vi "Engaging.vi"(6 "PID Cluster":T2={"L1 to L4 PID Cluster"={"L1 PID Gains"={"Kp"=0.005, "Kd"=0.5, "Ki"=0.0005}, "L2 PID Gains"={"Kp"=0.01, "Kd"=1.0, "Ki"=0.005}, "L3 PID Gains"={"Kp"=0.05, "Kd"=1.0, "Ki"=0.0005}, "L4 PID Gains"={"Kp"=0.1, "Kd"=0.1, "Ki"=0.0005}}, "Stage PID Cluster"={"Stage Z PID"={"Kp"=0.0005, "Kd"=0.001, "Ki"=0.0}, "Stage Y PID"={"Kp"=0.0003, "Kd"=0.01, "Ki"=0.0}, "Stage X PID"={"Kp"=0.0003, "Kd"=0.01, "Ki"=0.0}}, "OCT Z PID Gains"={"Kp"=0.0003, "Kd"=0.0001, "Ki"=0.01}}, 7 "Offset Home 2 RCM":dbl[](array[numeric])=[0.0, 0.0, 0.0, 0.0], 8 "error in":errorcluster, 9 "Engage Pt":dbl[](array[numeric])=[0.0, 0.0, 0.0, 0.0], 10 "Prev Posit Cluster":T3={"Prev L1 to L4 Posit"=[0.0, 0.0, 0.0, 0.0], "Prev Stage Posit"=[6.0, 6.0, 6.0], "Prev OCT Z Posit"=0.0}, 11 "FPGA VI Reference In":refnum<k20>) -> (0 "error out":errorcluster, 2 "Last Posit Cluster":T1={"Last L1 to L4 Posit"=[0.0, 0.0, 0.0, 0.0], "Last Stage Posit"=[6.0, 6.0, 6.0], "Last OCT Z Posit"=0.0}, 3 "FPGA VI Reference Out":refnum<k20>)   [LabVIEW 2016]
uses:
  <vilib>/Platform/TimedLoop/XDataNode/timing_clust.ctl
  <vilib>/Platform/TimedLoop/XDataNode/nitl_modes.ctl
  <vilib>/Platform/TimedLoop/XDataNode/wakeup.ctl
  Global Variables.vi
  <vilib>/platform/TimedLoop/XDataNode/XDataNode.xnode
  <vilib>/Platform/TimedLoop/XDataNode/XDNodeRunTimeDep.lvlib
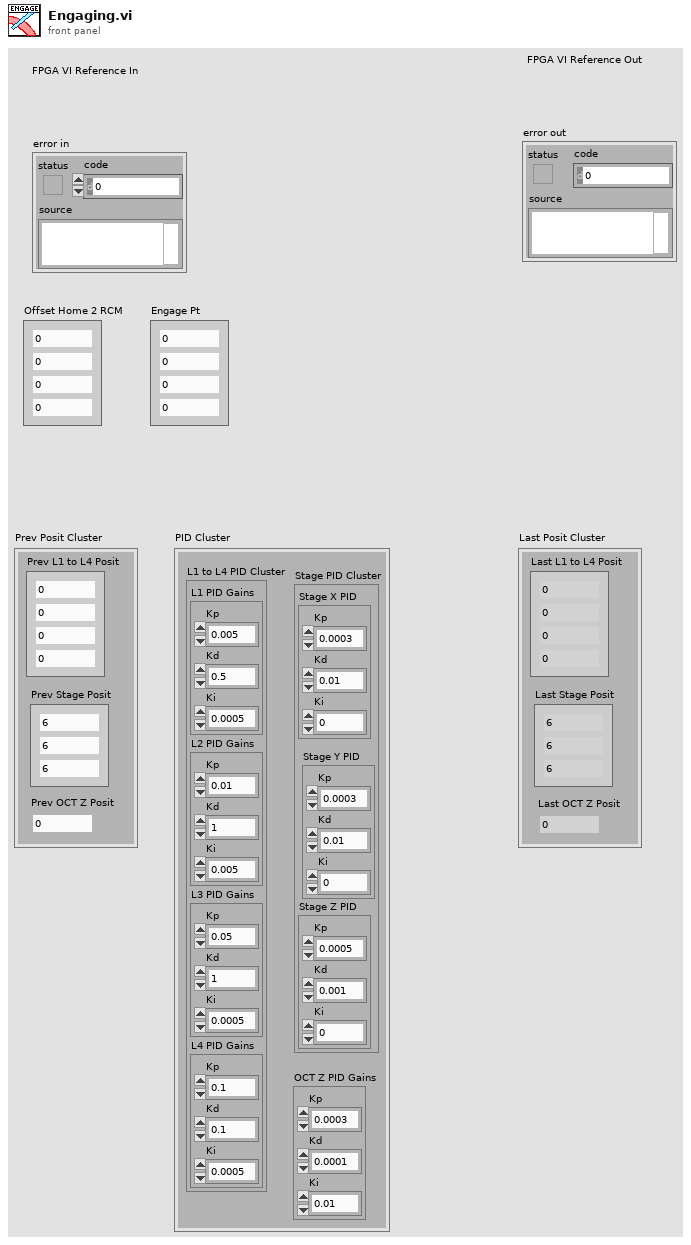
[diagram p1: front panel]
types:
  T1 = cluster{"Last L1 to L4 Posit":dbl[], "Last Stage Posit":dbl[], "Last OCT Z Posit":dbl}
  T2 = cluster{"L1 to L4 PID Cluster":cluster{"L1 PID Gains":cluster{"Kp":dbl, "Kd":dbl, "Ki":dbl}, "L2 PID Gains":cluster{"Kp":dbl, "Kd":dbl, "Ki":dbl}, "L3 PID Gains":cluster{"Kp":dbl, "Kd":dbl, "Ki":dbl}, "L4 PID Gains":cluster{"Kp":dbl, "Kd":dbl, "Ki":dbl}}, "Stage PID Cluster":cluster{"Stage Z PID":cluster{"Kp":dbl, "Kd":dbl, "Ki":dbl}, "Stage Y PID":cluster{"Kp":dbl, "Kd":dbl, "Ki":dbl}, "Stage X PID":cluster{"Kp":dbl, "Kd":dbl, "Ki":dbl}}, "OCT Z PID Gains":cluster{"Kp":dbl, "Kd":dbl, "Ki":dbl}}
  T3 = cluster{"Prev L1 to L4 Posit":dbl[], "Prev Stage Posit":dbl[], "Prev OCT Z Posit":dbl}
  T4 = cluster{"Stop Vacuum":bool, "Vacuum Force":i8, "Max Limit [mmHg]":dbl, "Slide in":i8, "Irrigation?":bool}
  T5 = typedef "XDNodeRunTimeDep.lvlib/timing_clust.ctl" = cluster{"Expected End [f-1]":u64, "Actual End [f-1]":u64, "Finished Late? [f-1]":bool, "Expected End [i-1]":u64, "Actual End [i-1]":u64, "Finished Late? [i-1]":bool, "Expected Start [i]":u64, "Actual Start [i]":u64, "Expected Start [f]":u64, "Actual Start [f]":u64, "Source Name":string, "Structure Name":string, "Period":i64, "Deadline":i64, "Offset":i64, "Start":i64, "Priority":i32, "Timeout":i32, "Mode":T6, "Wakeup Reason":T7, "Error":errorcluster, "Source Type":string, "Secondary Source Type":string, "Global End Time":u64, "Global Start Time":u64, "Frame Duration":u64, "Iteration Duration":u64, "Assigned CPU":i32, "I/O Scan Engine Mode":u32}
  T6 = typedef "XDNodeRunTimeDep.lvlib/nitl_modes.ctl" = enum32{"No Change", "Process missed periods, maintain original phase", "Discard missed periods, maintain original phase", "Process missed periods, ignore original phase", "Discard missed periods, ignore original phase"}
  T7 = typedef "XDNodeRunTimeDep.lvlib/wakeup.ctl" = enum32{"Normal", "Aborted", "Asynchronous wakeup", "Timing source error", "Timed loop error", "Timeout"}
  T8 = cluster{"Stage Z PID":cluster{"Kp":dbl, "Kd":dbl, "Ki":dbl}, "Stage Y PID":cluster{"Kp":dbl, "Kd":dbl, "Ki":dbl}, "Stage X PID":cluster{"Kp":dbl, "Kd":dbl, "Ki":dbl}}
  T9 = cluster{"L1 PID Gains":cluster{"Kp":dbl, "Kd":dbl, "Ki":dbl}, "L2 PID Gains":cluster{"Kp":dbl, "Kd":dbl, "Ki":dbl}, "L3 PID Gains":cluster{"Kp":dbl, "Kd":dbl, "Ki":dbl}, "L4 PID Gains":cluster{"Kp":dbl, "Kd":dbl, "Ki":dbl}}
  T10 = cluster{"Accurus button":bool[], "Accurus engaged?":bool, "Vacuum Force":i32, "Accurus Ch. A Vout":dbl, "Accurus Ch. B Vout":dbl, "Irrigation engaged?":bool}
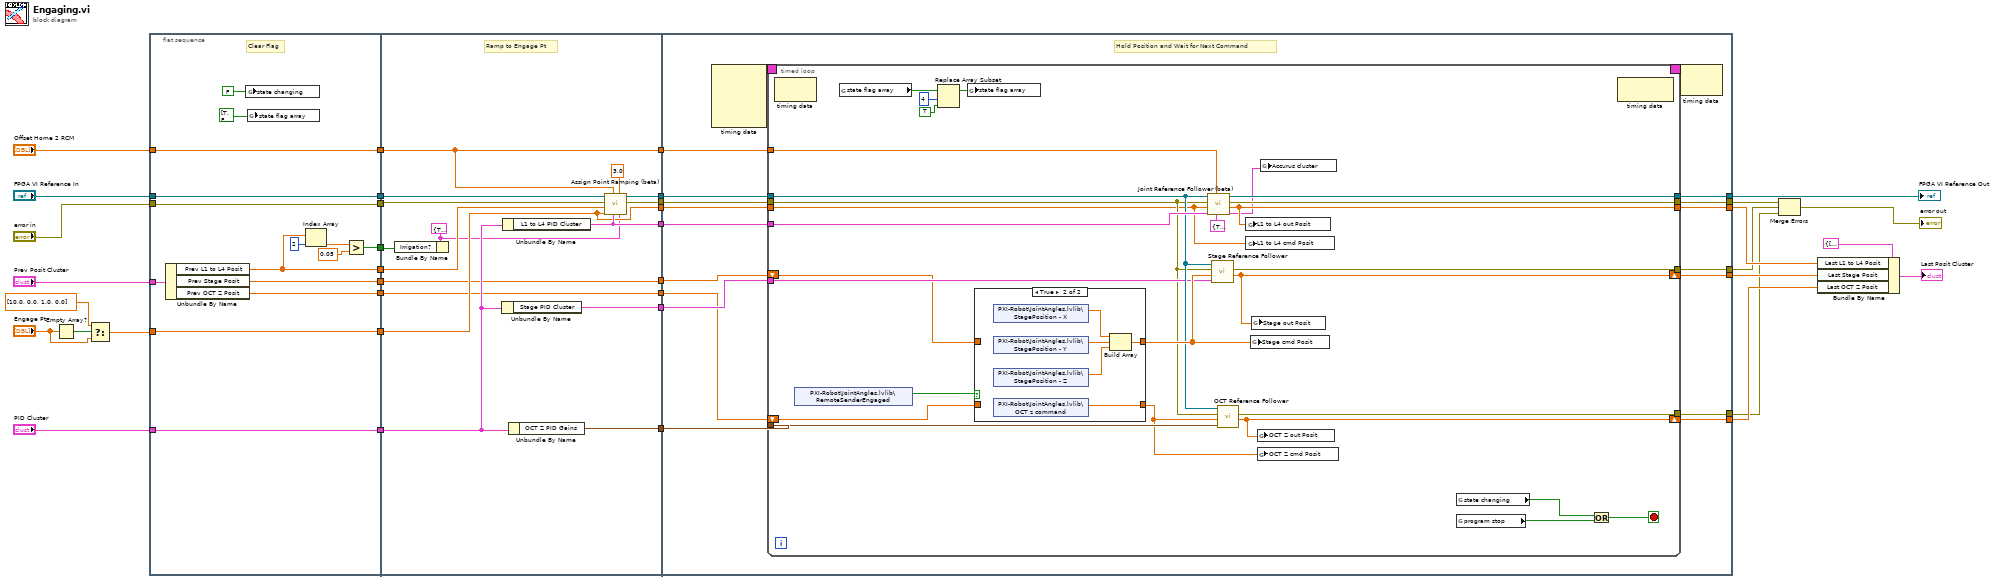
[diagram p0: block diagram]
diagram:
  n1 = Empty Array?(array="Engage Pt") -> (empty?=w29:bool)
  n2 = Select(t=dbl[] [10.0, 0.0, 1.0, 0.0] ("First Trk Pt 2"), s=w29, f="Engage Pt") -> (s? t:f=w26:dbl[])
  n3 = flat-sequence {
    tunnel: [w50] -> w37
    tunnel: "FPGA VI Reference In" -> [w50]
    tunnel: "error in" -> [w49]
    tunnel: [w49] -> w36
    tunnel: [w39] -> w35
    tunnel: "PID Cluster" -> [w47]
    tunnel: "Offset Home 2 RCM" -> [w48]
    tunnel: [w48] -> w33
    tunnel: [w43] -> w31
    tunnel: w26 -> [w43]
    tunnel: [w47] -> w19
    tunnel: "Prev Posit Cluster" -> [w46]
    tunnel: [w45] -> w5
    tunnel: [w44] -> w2
    tunnel: [w38] -> w1
    tunnel: w37 -> [w68]
    tunnel: w36 -> [w67]
    tunnel: w35 -> [w65]
    tunnel: w33 -> [w62]
    tunnel: w31 -> [w57]
    tunnel: [w64] -> w30
    tunnel: [w57] -> w25
    tunnel: [w63] -> w24
    tunnel: [w62] -> w23
    tunnel: [w61] -> w22
    tunnel: w19 -> [w59]
    tunnel: [w60] -> w18
    tunnel: [w58] -> w17
    tunnel: w5 -> [w56]
    tunnel: [w56] -> w4
    tunnel: [w55] -> w3
    tunnel: w2 -> [w55]
    tunnel: w1 -> [w54]
    tunnel: [w80] -> w13
    tunnel: [w79] -> w8
    tunnel: w30 -> [w83]
    tunnel: w25 -> [w82]
    tunnel: w24 -> [w84]
    tunnel: w23 -> [w71]
    tunnel: w22 -> [w81]
    tunnel: [w78] -> w20
    tunnel: [w77] -> w21
    tunnel: w18 -> [w76]
    tunnel: w17 -> [w75]
    tunnel: [w74] -> w14
    tunnel: [w73] -> w7
    tunnel: [w72] -> w6
    tunnel: w4 -> [w70]
    tunnel: w3 -> [w69]
    frame #0 {
      # "Clear Flag"
      n4 = Unbundle By Name(w46) -> ("Prev L1 to L4 Posit"=w39:dbl[], "Prev Stage Posit"=w45:dbl[], "Prev OCT Z Posit"=w44:dbl)
      n5 = global write "Global Variables.vi" "state changing"(FALSE ("state changing")) -> ()
      n6 = global write "Global Variables.vi" "state flag array"(bool[] [TRUE, FALSE, FALSE, FALSE, FALSE, FALSE, FALSE, FALSE, FALSE] ("state flag array")) -> ()
      n7 = Index Array(array=w39, index=2) -> (element=w41:dbl)
      n8 = Greater?(x=w41, y=0.05) -> (0:w38:bool)
    }
    frame #1 {
      w53 = T4 {"Stop Vacuum"=TRUE, "Vacuum Force"=0, "Max Limit [mmHg]"=600.0, "Slide in"=0, "Irrigation?"=FALSE} ("Accurus Ctrl Cluster")
      # "Ramp to Engage Pt"
      n9 = Bundle By Name(cluster=w53, "Irrigation?"=w54) -> ()  [unwired: 1 out]
      n10 = Unbundle By Name(w59) -> ("Stage PID Cluster"=w60:T8)
      n11 = Unbundle By Name(w59) -> ("L1 to L4 PID Cluster"=w61:T9)
      n12 = Unbundle By Name(w59) -> ("OCT Z PID Gains"=w58:cluster{"Kp":dbl, "Kd":dbl, "Ki":dbl})
      n13 = call "Assign Point Ramping (beta).vi"("Accurus Ctrl Cluster"=w53, "Ramp Time [sec]"=3.0, "L1 to L4 PID Cluster"=w61, "Offset Home2RCM"=w62, "Destination Posit Array [mm]"=w57, "Previous Posit Array"=w65, "error in"=w67, "FPGA VI Reference In"=w68) -> ("error out"=w64:errorcluster, "FPGA VI Reference Out"=w63:refnum<k20>)  [unwired: 1 in, 1 out]
    }
    frame #2 {
      # "Hold Position and Wait for Next Command"
      n14 = node-c288() -> (w86:T5)  [unwired: 4 in]
      n15 = timed-loop {
        timing: w86 -> [_]
        timing-out: [_] -> w85
        tunnel: w84 -> [w103]
        tunnel: w83 -> [w95]
        tunnel: w71 -> [w109]
        tunnel: w82 -> [w89]
        tunnel: w81 -> [w108]
        tunnel: [w107] -> w80
        tunnel: [w106] -> w79
        tunnel: [w101] -> w78
        tunnel: w76 -> [w100]
        tunnel: w75 -> [w99]
        tunnel: [w94] -> w73
        tunnel: [w93] -> w72
        shift-right: [w104] -> w77
        shift-left: w70 -> [w91]
        shift-right: [w98] -> w74
        shift-left: w69 -> [w90]
        stop <- w96 stop-if-true
        n16 = node-c288() -> ()  [unwired: 1 in, 1 out]
        n17 = shared-variable "PXI-Robot\\JointAngles.lvlib\\RemoteSenderEngaged"() -> (w92:bool)  [unwired: 1 in, 1 out]
        n18 = global read "Global Variables.vi" "state flag array"() -> (w113:bool[])
        n19 = Replace Array Subset(array=w113, new element=TRUE ("new element/subarray"), index=4) -> (w112:bool[])
        n20 = global write "Global Variables.vi" "state flag array"(w112) -> ()
        n21 = case shown="True" w92 {
          tunnel: [w116 w118] -> w105
          tunnel: [w115 w117] -> w97
          tunnel: w91 -> [w116 _]
          tunnel: w90 -> [w115 _]
          frame False {
            # "Hold Position if not Engaged"
          }
          frame True {
            n22 = shared-variable "PXI-Robot\\JointAngles.lvlib\\StagePosition - X"() -> (w121:dbl)  [unwired: 1 in, 1 out]
            n23 = shared-variable "PXI-Robot\\JointAngles.lvlib\\StagePosition - Y"() -> (w120:dbl)  [unwired: 1 in, 1 out]
            n24 = shared-variable "PXI-Robot\\JointAngles.lvlib\\StagePosition - Z"() -> (w119:dbl)  [unwired: 1 in, 1 out]
            n25 = shared-variable "PXI-Robot\\JointAngles.lvlib\\OCT z command"() -> (w117:dbl)  [unwired: 1 in, 1 out]
            n26 = Build Array(w121, w120, w119) -> (w118:dbl[])
          }
        }
        n27 = call "Joint Reference Follower (beta).vi"("Accurus Ctrl Cluster"=T4 {"Stop Vacuum"=TRUE, "Vacuum Force"=0, "Max Limit [mmHg]"=600.0, "Slide in"=0, "Irrigation?"=TRUE}, "Offset Home2RCM [deg/mm]"=w109, "PID Ctrl Cluster"=w108, "Ref Array [deg/mm]"=w89, "error in"=w95, "FPGA VI Reference In"=w103) -> ("Accurus Output Cluster"=w88:T10, "Output Posit Array [deg/mm]"=w101:dbl[], "error out"=w106:errorcluster, "FPGA VI Reference Out"=w107:refnum<k20>)  [unwired: 2 in]
        n28 = call "Stage Reference Follower.vi"("Stage PID Cluster"=w100, "Stage cmd Posit [mm]"=w105, "error in"=w95, "FPGA VI Reference In"=w103) -> ("Stage out Posit [mm]"=w104:dbl[], "error out"=w94:errorcluster)  [unwired: 5 in, 1 out]
        n29 = call "OCT Reference Follower.vi"("OCT Z PID Gains"=w99, "OCT  Z cmd Posit [mm]"=w97, "error in"=w95, "FPGA VI Reference In"=w103) -> ("OCT  Z out Posit [mm]"=w98:dbl, "error out"=w93:errorcluster)  [unwired: 5 in, 1 out]
        n30 = global write "Global Variables.vi" "L1 to L4 out Posit"(w101) -> ()
        n31 = global write "Global Variables.vi" "L1 to L4 cmd Posit"(w89) -> ()
        n32 = global write "Global Variables.vi" "Stage cmd Posit"(w105) -> ()
        n33 = global write "Global Variables.vi" "Stage out Posit"(w104) -> ()
        n34 = global write "Global Variables.vi" "OCT Z out Posit"(w98) -> ()
        n35 = global write "Global Variables.vi" "OCT Z cmd Posit"(w97) -> ()
        n36 = global write "Global Variables.vi" "Accurus cluster"(w88) -> ()
        n37 = global read "Global Variables.vi" "state changing"() -> (w114:bool)
        n38 = global read "Global Variables.vi" "program stop"() -> (w102:bool)
        n39 = Or(x=w114, y=w102) -> (x .or. y?=w96:bool)
        n40 = node-c288() -> ()  [unwired: 1 in, 1 out]
      }
      n41 = node-c288(w85) -> ()  [unwired: 1 out]
    }
  }
  n42 = Merge Errors(w8, w7, w6) -> (→"error out":errorcluster)
  n43 = Bundle By Name(cluster=T1 {"Last L1 to L4 Posit"=[0.0, 0.0, 0.0, 0.0], "Last Stage Posit"=[6.0, 6.0, 6.0], "Last OCT Z Posit"=0.0} ("Last Posit Cluster 2"), "Last L1 to L4 Posit"=w20, "Last Stage Posit"=w21, "Last OCT Z Posit"=w14) -> (→"Last Posit Cluster":T1)
  "FPGA VI Reference Out" <- w13
